vi "WPI_CounterSetExternalReset.vi"(8 "error in (no error)":errorcluster, 9 "IndexActiveHigh":bool=TRUE, 10 "IndexSource":T3={"DevStatus"={"status"=FALSE, "code"=0, "source"=""}, "AnalogTriggerMode?"=FALSE, "DigitalMode"={"DIO Channel"=enum."DIO 1"}, "AnalogTriggerMode"={"AnalogTriggerIndex"=enum."Trig 0", "OutputType"=enum."InWindow"}}, 11 "CounterDevRef in":T1) -> (0 "error out":errorcluster, 3 "CounterDevRef out":T1)   [LabVIEW 2017]
doc: "This software is licensed. Open the labview\\readme\\WPI Robotics Library Open Source License.txt file for more information."
uses:
  <vilib>/Rock Robotics/SystemInterfaces/CounterEncoderSourceConvertion/FPGA_CounterEncoderSourceConvertionLVSourceType.ctl
  <vilib>/Rock Robotics/SystemInterfaces/DIO/FPGA_DIODigitalSourceChannel.ctl
  <vilib>/Rock Robotics/SystemInterfaces/AnalogTrigger/FPGA_AnalogTriggerIndex.ctl
  <vilib>/Rock Robotics/SystemInterfaces/AnalogTrigger/FPGA_AnalogTriggerOutType.ctl
  <vilib>/Rock Robotics/WPI/Counter/WPI_CounterDevRef.ctl
  <vilib>/Rock Robotics/SystemInterfaces/Counter/FPGA_CounterCtrSystemIndex.ctl
  <vilib>/Rock Robotics/SystemInterfaces/Counter/FPGA_CounterERRInvalidResource.vi
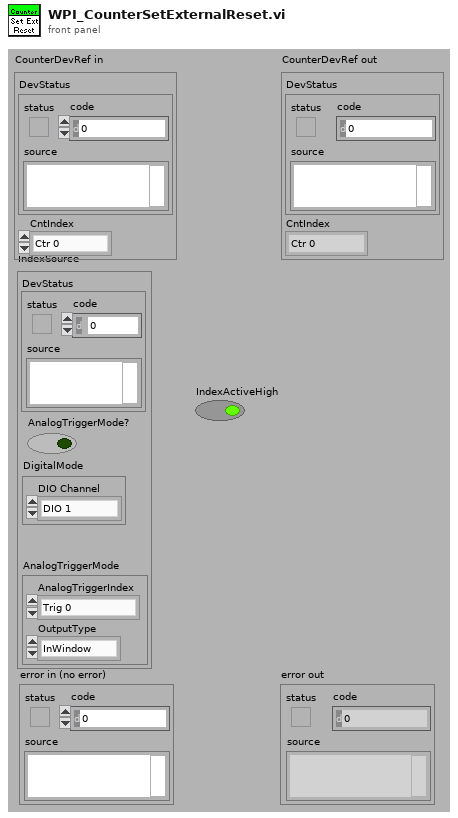
[diagram p1: front panel]
types:
  T1 = typedef "WPI_CounterDevRef.ctl" = cluster{"DevStatus":errorcluster, "CntIndex":T2}
  T2 = typedef "FPGA_CounterCtrSystemIndex.ctl" = enum8{"Ctr 0", "Ctr 1", "Ctr 2", "Ctr 3", "Ctr 4", "Ctr 5", "Ctr 6", "Ctr 7", "Invalid"}
  T3 = typedef "FPGA_CounterEncoderSourceConvertionLVSourceType.ctl" = cluster{"DevStatus":errorcluster, "AnalogTriggerMode?":bool, "DigitalMode":cluster{"DIO Channel":T4}, "AnalogTriggerMode":cluster{"AnalogTriggerIndex":T5, "OutputType":T6}}
  T4 = typedef "FPGA_DIODigitalSourceChannel.ctl" = enum8{"DIO 0", "DIO 1", "DIO 2", "DIO 3", "DIO 4", "DIO 5", "DIO 6", "DIO 7", "DIO 8", "DIO 9", "DIO MXP 0", "DIO MXP 1", "DIO MXP 2", "DIO MXP 3", "DIO MXP 4", "DIO MXP 5", "DIO MXP 6", "DIO MXP 7", "DIO MXP 8", "DIO MXP 9", "DIO MXP 10", "DIO MXP 11", "DIO MXP 12", "DIO MXP 13", "DIO MXP 14", "DIO MXP 15", "Disabled"}
  T5 = typedef "FPGA_AnalogTriggerIndex.ctl" = enum8{"Trig 0", "Trig 1", "Trig 2", "Trig 3", "Trig 4", "Trig 5", "Trig 6", "Trig 7", "Invalid"}
  T6 = typedef "FPGA_AnalogTriggerOutType.ctl" = enum16{"InWindow", "TriggerState", "Rising", "Falling"}
  T7 = typedef "FPGA_CounterCtrDevRef.ctl" = cluster{"DevStatus":errorcluster, "CntIndex":T2}
  T8 = typedef "FPGA_CounterCtrEdgeDetectionType.ctl" = cluster{"Master Mode":enum16{"Edge Detection", "Semi Period Mode", "Pulse Length Mode", "External Direction"}, "UpChannel":enum16{"Rising Edge", "Falling Edge", "Raising & Falling Edge", "Disabled"}, "DownChannel":enum16{"Rising Edge", "Falling Edge", "Raising & Falling Edge", "Disabled"}, "High/Up":bool}
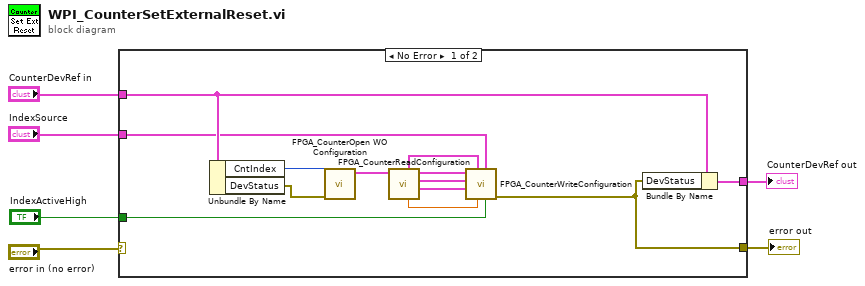
[diagram p0: block diagram]
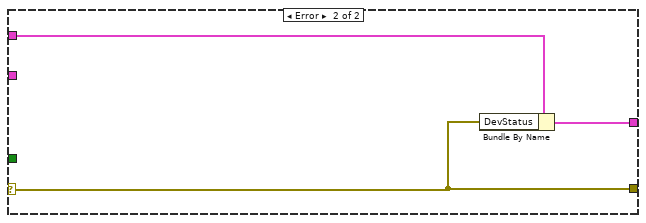
[diagram p2: hidden frame]
diagram:
  n1 = case shown="No Error" "error in (no error)" {
    selector: "error in (no error)" -> [_ w20]
    tunnel: "CounterDevRef in" -> [w11 w22]
    tunnel: [w19 w21] -> w5
    tunnel: [w7 w20] -> w3
    tunnel: "IndexSource" -> [w8 _]
    tunnel: "IndexActiveHigh" -> [w9 _]
    frame No Error {
      n2 = Unbundle By Name(w11) -> ("CntIndex"=w18:T2, "DevStatus"=w13:errorcluster)
      n3 = call <vilib>:"FPGA_CounterOpen WO Configuration.vi"("error in"=w13, "CntIndex"=w18) -> ("Ctr Ref"=w17:T7)  [unwired: 1 in, 8 out]
      n4 = call <vilib>:"FPGA_CounterReadConfiguration.vi"("Ctr Ref in"=w17) -> ("DownSource"=w10:T3, "UpSource"=w15:T3, "Ctr Ref out"=w16:T7, "GTSDirThreshold"=w14:sgl, "EdgeType"=w12:T8)  [unwired: 1 in, 5 out]
      n5 = call <vilib>:"FPGA_CounterWriteConfiguration.vi"("IndexActiveHigh"=w9, "IndexSource"=w8, "GTSDirThreshold"=w14, "EdgeType"=w12, "DownSource"=w10, "UpSource"=w15, "Ctr Ref in"=w16) -> ("error out"=w7:errorcluster)  [unwired: 2 in, 2 out]
      n6 = Bundle By Name(cluster=w11, "DevStatus"=w7) -> (w19:T1)
    }
    frame Error {
      n7 = Bundle By Name(cluster=w22, "DevStatus"=w20) -> (w21:T1)
    }
  }
  "CounterDevRef out" <- w5
  "error out" <- w3
